vi "Connect.vi"(8 "error in (no error)":errorcluster, 11 "FTPProtocol in":refnum<class "FTPProtocol.lvclass">) -> (0 "error out":errorcluster, 1 "Connected?":bool=TRUE, 3 "FTPProtocol out":refnum<class "FTPProtocol.lvclass">)   [LabVIEW 2017, in "FileSync -- FTP.lvlib" / "FTPProtocol.lvclass"]
uses:
  FTPProtocol.lvclass
  FTPProtocol.lvclass/FTPProtocol.ctl
  FTPConfig/FTPConfig.lvclass/FTPConfig.ctl
  FTPConfig/Read config.vi
  _support/FTP Toolkit/FTP Class/FTP.lvclass
  FTPConfig/FTPConfig.lvclass
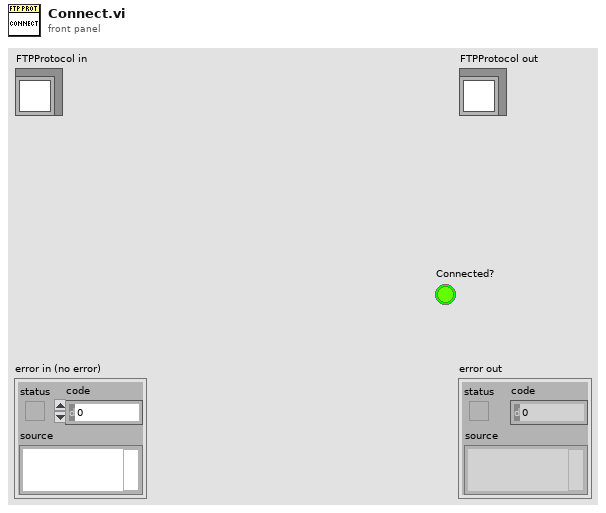
[diagram p1: front panel]
types:
  T1 = typedef "FileSync -- FTP.lvlib/FTPConfig.lvclass/Def-FTP Server Info.vi" = cluster{"address":string, "remote port":u16, "userName":string, "passWord":string, "RootDir":string}
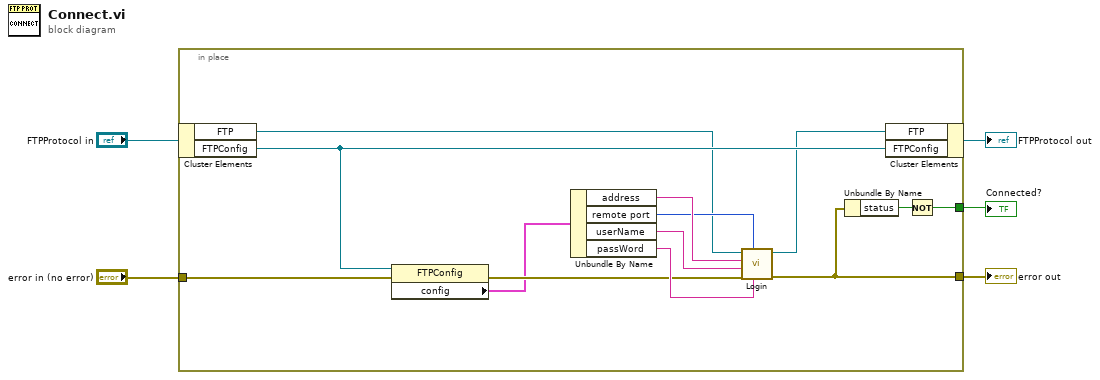
[diagram p0: block diagram]
diagram:
  n1 = in-place {
    in-place-border: "error in (no error)" -> [w14]
    in-place-border: [w7] -> w4
    in-place-border: [w6] -> w1
    n2 = in-place-cluster #1("FTPProtocol in") -> ("FTP"=w9:refnum<class "FTP.lvclass">, "FTPConfig"=w11:refnum<class "FTPConfig.lvclass">)
    n3 = property class="FTPConfig"(reference=w11, error in=w14) -> (error out=w13:errorcluster, "config"=w12:T1)  [unwired: 1 out]
    n4 = Unbundle By Name(w12) -> ("address"=w18:string, "remote port"=w17:u16, "userName"=w16:string, "passWord"=w15:string)
    n5 = call "Login.vi"("passWord"=w15, "remote port (21)"=w17, "error in (no error)"=w13, "userName"=w16, "address"=w18, "FTP in"=w9) -> ("error out"=w7:errorcluster, "FTP out"=w10:refnum<class "FTP.lvclass">)  [unwired: 4 in]
    n6 = Unbundle By Name(w7) -> ("status"=w8:bool)
    n7 = in-place-cluster #1("FTP"=w10, "FTPConfig"=w11) -> (→"FTPProtocol out":refnum<class "FTPProtocol.lvclass">)
    n8 = Not(x=w8) -> (.not. x?=w6:bool)
  }
  "error out" <- w4
  "Connected?" <- w1
